vi "GetTextFromBoolCtrl.vi"(11 "bool ref":refnum<vi>) -> (3 "result":string)   [LabVIEW 2018, in "Library-Ctrl.lvlib"]
uses:
  Library-Ctrl.lvlib
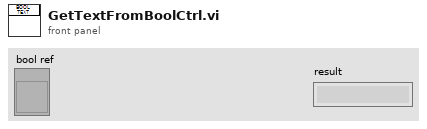
[diagram p1: front panel]
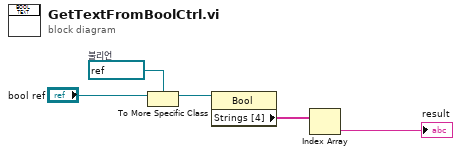
[diagram p0: block diagram]
diagram:
  w4 = refnum<vi> refnum  # 불리언
  n1 = To More Specific Class(target class=w4, reference="bool ref") -> (specific class reference=w3:refnum<vi>)  [unwired: 1 in, 1 out]
  n2 = property class="Bool"(reference=w3) -> ("Strings [4]"=w2:string[])  [unwired: 1 in, 2 out]
  n3 = Index Array(array=w2) -> (element=→"result":string)  [unwired: 1 in]
